vi "Split Path Segments.vi"(8 "error in (no error)":errorcluster, 11 "Base Path in":path) -> (0 "error out":errorcluster, 1 "Constant Path":bool, 2 "Path Segments":T1[](array[typedef]), 3 "Base Path out":path)   [LabVIEW 2012, in "Waveform Data Logger Shared.lvlib" / "Log File Specification.lvclass"]
doc: "Split the path into path segments, which are either raw strings or tags that get evaluated when the instance path is built."
uses:
  Log File Specification.lvclass
  Path Segment.ctl
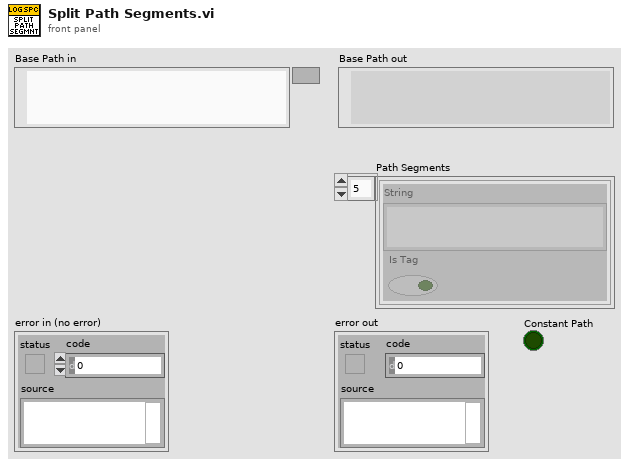
[diagram p1: front panel]
types:
  T1 = typedef "Waveform Data Logger Shared.lvlib/Log File Specification.lvclass/Path Segment.ctl" = cluster{"String":string, "Is Tag":bool}
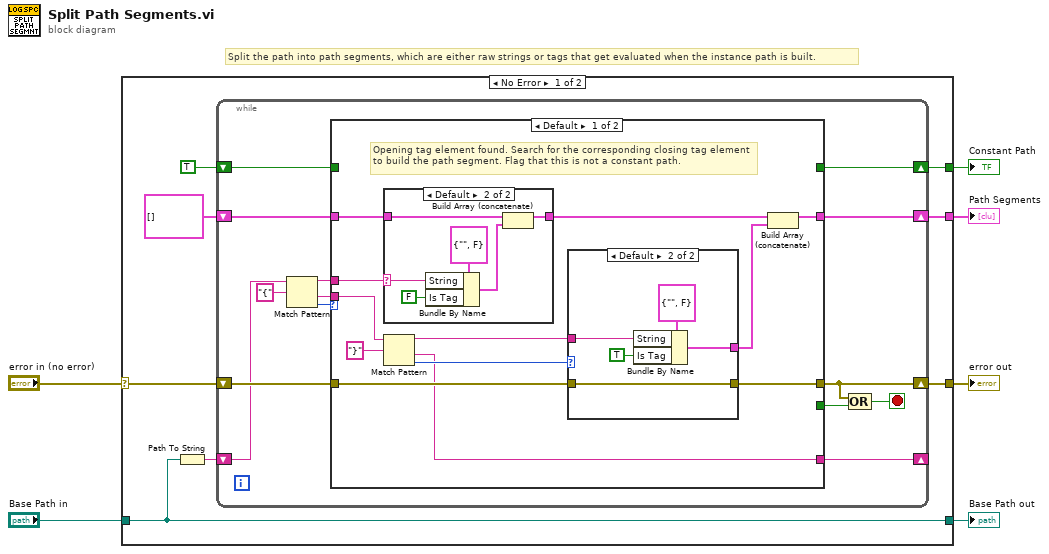
[diagram p0: block diagram]
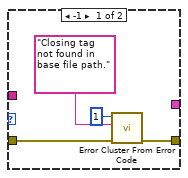
[diagram p3: hidden frame]
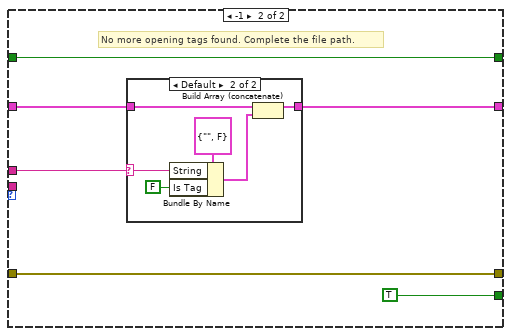
[diagram p4: hidden frame]
diagram:
  # "Split the path into path segments, which are either raw strings or tags that get evaluated when the instance path is built."
  n1 = case shown="No Error" "error in (no error)" {
    selector: "error in (no error)" -> [w10 w71]
    tunnel: "Base Path in" -> [w9 w70]
    tunnel: [w14 _] -> w5
    tunnel: [w12 w71] -> w4
    tunnel: [w9 w70] -> w2
    tunnel: [w7 _] -> w1
    frame No Error {
      n2 = Path To String(path=w9) -> (string=w11:string)
      n3 = while {
        shift-right: [w21] -> _
        shift-left: w11 -> [w26]
        shift-right: [w19] -> w12
        shift-left: w10 -> [w27]
        shift-right: [w16] -> w14
        shift-left: T1[] [] -> [w17]
        shift-right: [w15] -> w7
        shift-left: TRUE -> [w28]
        stop <- w20 stop-if-true
        n4 = Match Pattern(string=w26, regular expression="{" ("Open Tag Element (\"{\")")) -> (before substring=w22:string, after substring=w23:string, offset past match=w25:i32)  [unwired: 1 in, 1 out]
        n5 = case shown="Default" w25 {
          tunnel: [_ TRUE] -> w24
          tunnel: w23 -> [w38 _]
          tunnel: w22 -> [w30 w58]
          tunnel: [w37 _] -> w21
          tunnel: w27 -> [w39 w61]
          tunnel: [w36 w61] -> w19
          tunnel: w17 -> [w31 w60]
          tunnel: [w32 w59] -> w16
          tunnel: w28 -> [_ w57]
          tunnel: [_ w57] -> w15
          frame Default {
            # "Opening tag element found. Search for the corresponding closing tag element to build the path segment. Flag that this is not a constant path."
            n6 = case shown="Default" w30 {
              selector: w30 -> [_ w43]
              tunnel: w31 -> [w41 w45]
              tunnel: [w41 w42] -> w29
              frame "" {
              }
              frame Default {
                n7 = Bundle By Name(cluster=T1 {"String"="", "Is Tag"=FALSE} ("Path Segment"), "String"=w43, "Is Tag"=FALSE) -> (w44:T1)
                n8 = Build Array (concatenate)(w45, w44) -> (w42:T1[])
              }
            }
            n9 = Match Pattern(string=w38, regular expression="}" ("Close Tag Element (\"}\")")) -> (before substring=w35:string, after substring=w37:string, offset past match=w40:i32)  [unwired: 1 in, 1 out]
            n10 = case shown="Default" w40 {
              tunnel: w39 -> [w51 w56]
              tunnel: [w50 w56] -> w36
              tunnel: w35 -> [_ w53]
              tunnel: [_ w52] -> w33
              frame -1 {
                n11 = call <vilib>:"Error Cluster From Error Code.vi"("error in (no error)"=w51, "error message (\"\")"="Closing tag not found in base file path.", "error code (0)"=1) -> ("error out"=w50:errorcluster)  [unwired: 6 in]
              }
              frame Default {
                n12 = Bundle By Name(cluster=T1 {"String"="", "Is Tag"=FALSE} ("Path Segment"), "String"=w53, "Is Tag"=TRUE) -> (w52:T1)
              }
            }
            n13 = Build Array (concatenate)(w29, w33) -> (w32:T1[])
          }
          frame -1 {
            # "No more opening tags found. Complete the file path."
            n14 = case shown="Default" w58 {
              selector: w58 -> [_ w65]
              tunnel: w60 -> [w63 w67]
              tunnel: [w63 w64] -> w59
              frame "" {
              }
              frame Default {
                n15 = Bundle By Name(cluster=T1 {"String"="", "Is Tag"=FALSE} ("Path Segment"), "String"=w65, "Is Tag"=FALSE) -> (w66:T1)
                n16 = Build Array (concatenate)(w67, w66) -> (w64:T1[])
              }
            }
          }
        }
        n17 = Compound Arithmetic op=OR(w19, w24) -> (w20:bool)
      }
    }
    frame Error {
    }
  }
  "Path Segments" <- w5
  "error out" <- w4
  "Base Path out" <- w2
  "Constant Path" <- w1
